vi "BioFeedback20(simple load data).vi"() -> ()   [LabVIEW 2016]
doc: "Use this template to build a producer/consumer design pattern. Use this template when you need to execute a process, such as data analysis, when a data source, such as a triggered acquisition, produces data at an uneven rate and you need to execute the process when the data becomes available."
uses:
  customSubVIs/8ChanWfmArray.ctl
  <vilib>/Utility/file.llb/Write Delimited Spreadsheet (string).vi
  <vilib>/Waveform/WDTFileIO.llb/Export Waveforms To Spreadsheet File (1D).vi
panel:
  in  "enableSave":bool caption="No Save      Save"
  in  "barOrGraph":bool=TRUE caption="Graph (under construction)       Bar"
  in  "Trial comment":string
  out "Collecting Data":bool
  in  "Display Min":dbl
  in  "Display Max":dbl=100.0
  in  "log filepath":path
  out "TrialStartTime":timestamp
  in  "Trial Duration (s)":dbl=3.0
  out "Trial Number":dbl
  in  "Session Name":string="Test"
  out "loopTime":dbl=30.0 caption="Upper Cut-Off"
  in  "trial display data":path
  out "Disp Data":cluster{"queue out":refnum<queue>, dbl, dbl}[](array[cluster])
  in  "Target Percentage":dbl=10.0
  out "DisplayActivation":dbl
  out "DisplayBarActivation":dbl(slide) caption="Percent Activation" max=1.0 scale=0.0..100.0
  in  "EMG Channel To Display":dbl=1.0
  out "MVC Data":cluster{"queue out":refnum<queue>, dbl, dbl}[](array[cluster])
  out "Trial Name":string="Test"
  in  "Data Directory":path=path "C:/Users/Tinggroup/Desktop/EMG Biofeedback System/LabviewFiles/Data"
  out "GetMaxStartTime":timestamp
  in  "MVC Number":dbl=1.0
  in  "SecondsToAcquireMax":dbl=3.0
  in  "Frames Per Second":dbl=30.0 caption="Upper Cut-Off"
  in  "EMG Input Device\nProduct Type":string="USB-6009"
  out "raw data":dynamicdata(graph)
  out "dispSize":dbl=20.0 caption="Lower Cut-Off"
  out "mvcSize":dbl=300.0 caption="Upper Cut-Off"
  in  "MVC Window Size (s)":dbl=0.5
  in  "Display Window Size (s)":dbl=0.5
  in  "MVC Raw Path":path
  in  "trial raw data":path
  in  "trial filtered data":path
  in  "MVC Filtered Path":path
  in  "Sample rate (Hz)":dbl=1000.0 caption="Upper Cut-Off"
  out "fps":dbl=20.0 caption="Lower Cut-Off"
  out "rate":dbl=300.0 caption="Upper Cut-Off"
  in  "Set Parameters":bool
  out "lower":dbl=20.0 caption="Lower Cut-Off"
  out "upper":dbl=300.0 caption="Upper Cut-Off"
  in  "Lower Cut-Off":dbl=20.0
  in  "Upper Cut-Off":dbl=500.0
  in  "Mark":bool
  in  "End Trial":bool
  in  "Reset MVC":bool
  in  "Get MVC":bool
  in  "StartTrial":bool
  out "State":T1(ring)
  out "FilteredAndRectified":waveform(dbl)[](graph) caption="Filtered and Rectified"
  in  "stop":bool
  # "Filtering"
  # "Add trial name\nBEFORE beginning trial"
  # "Display Settings"
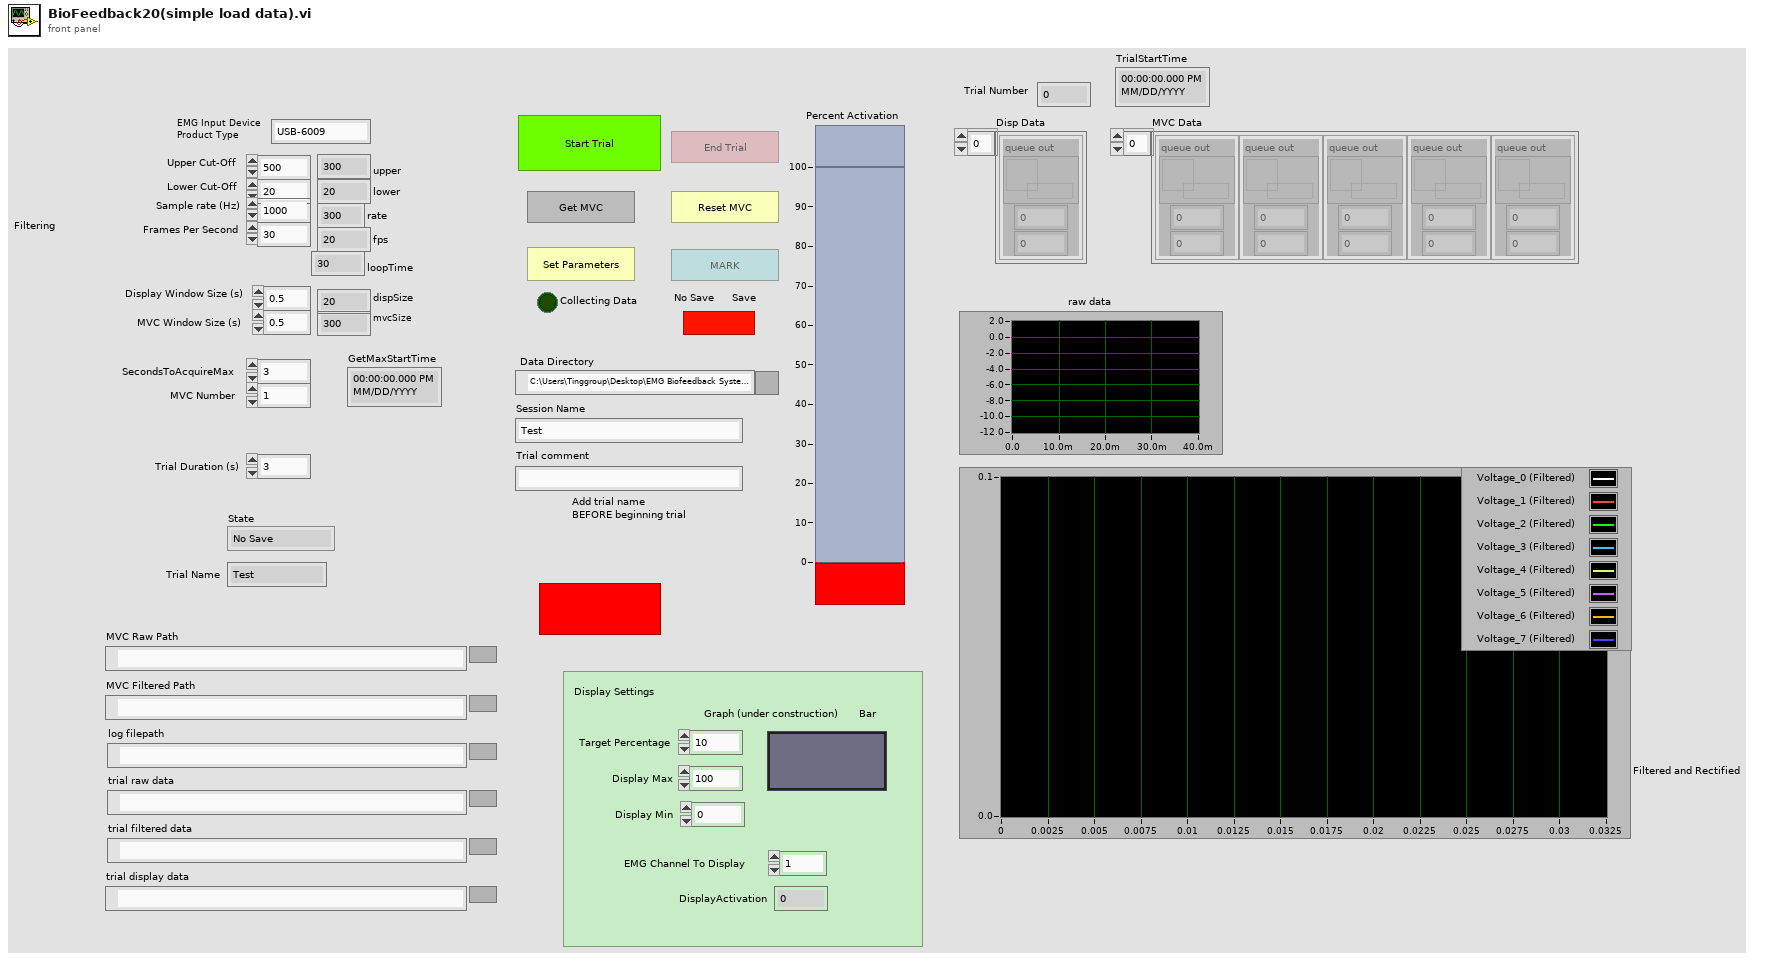
[diagram p1: front panel]
types:
  T1 = enum16{"No Save", "Acquiring Max", "Trial In Progress"}
  T2 = typedef "8ChanWfmArray.ctl" = waveform(dbl)[]
  T3 = enum8{"Enabled", "Disabled", "Disabled and Grayed Out"}
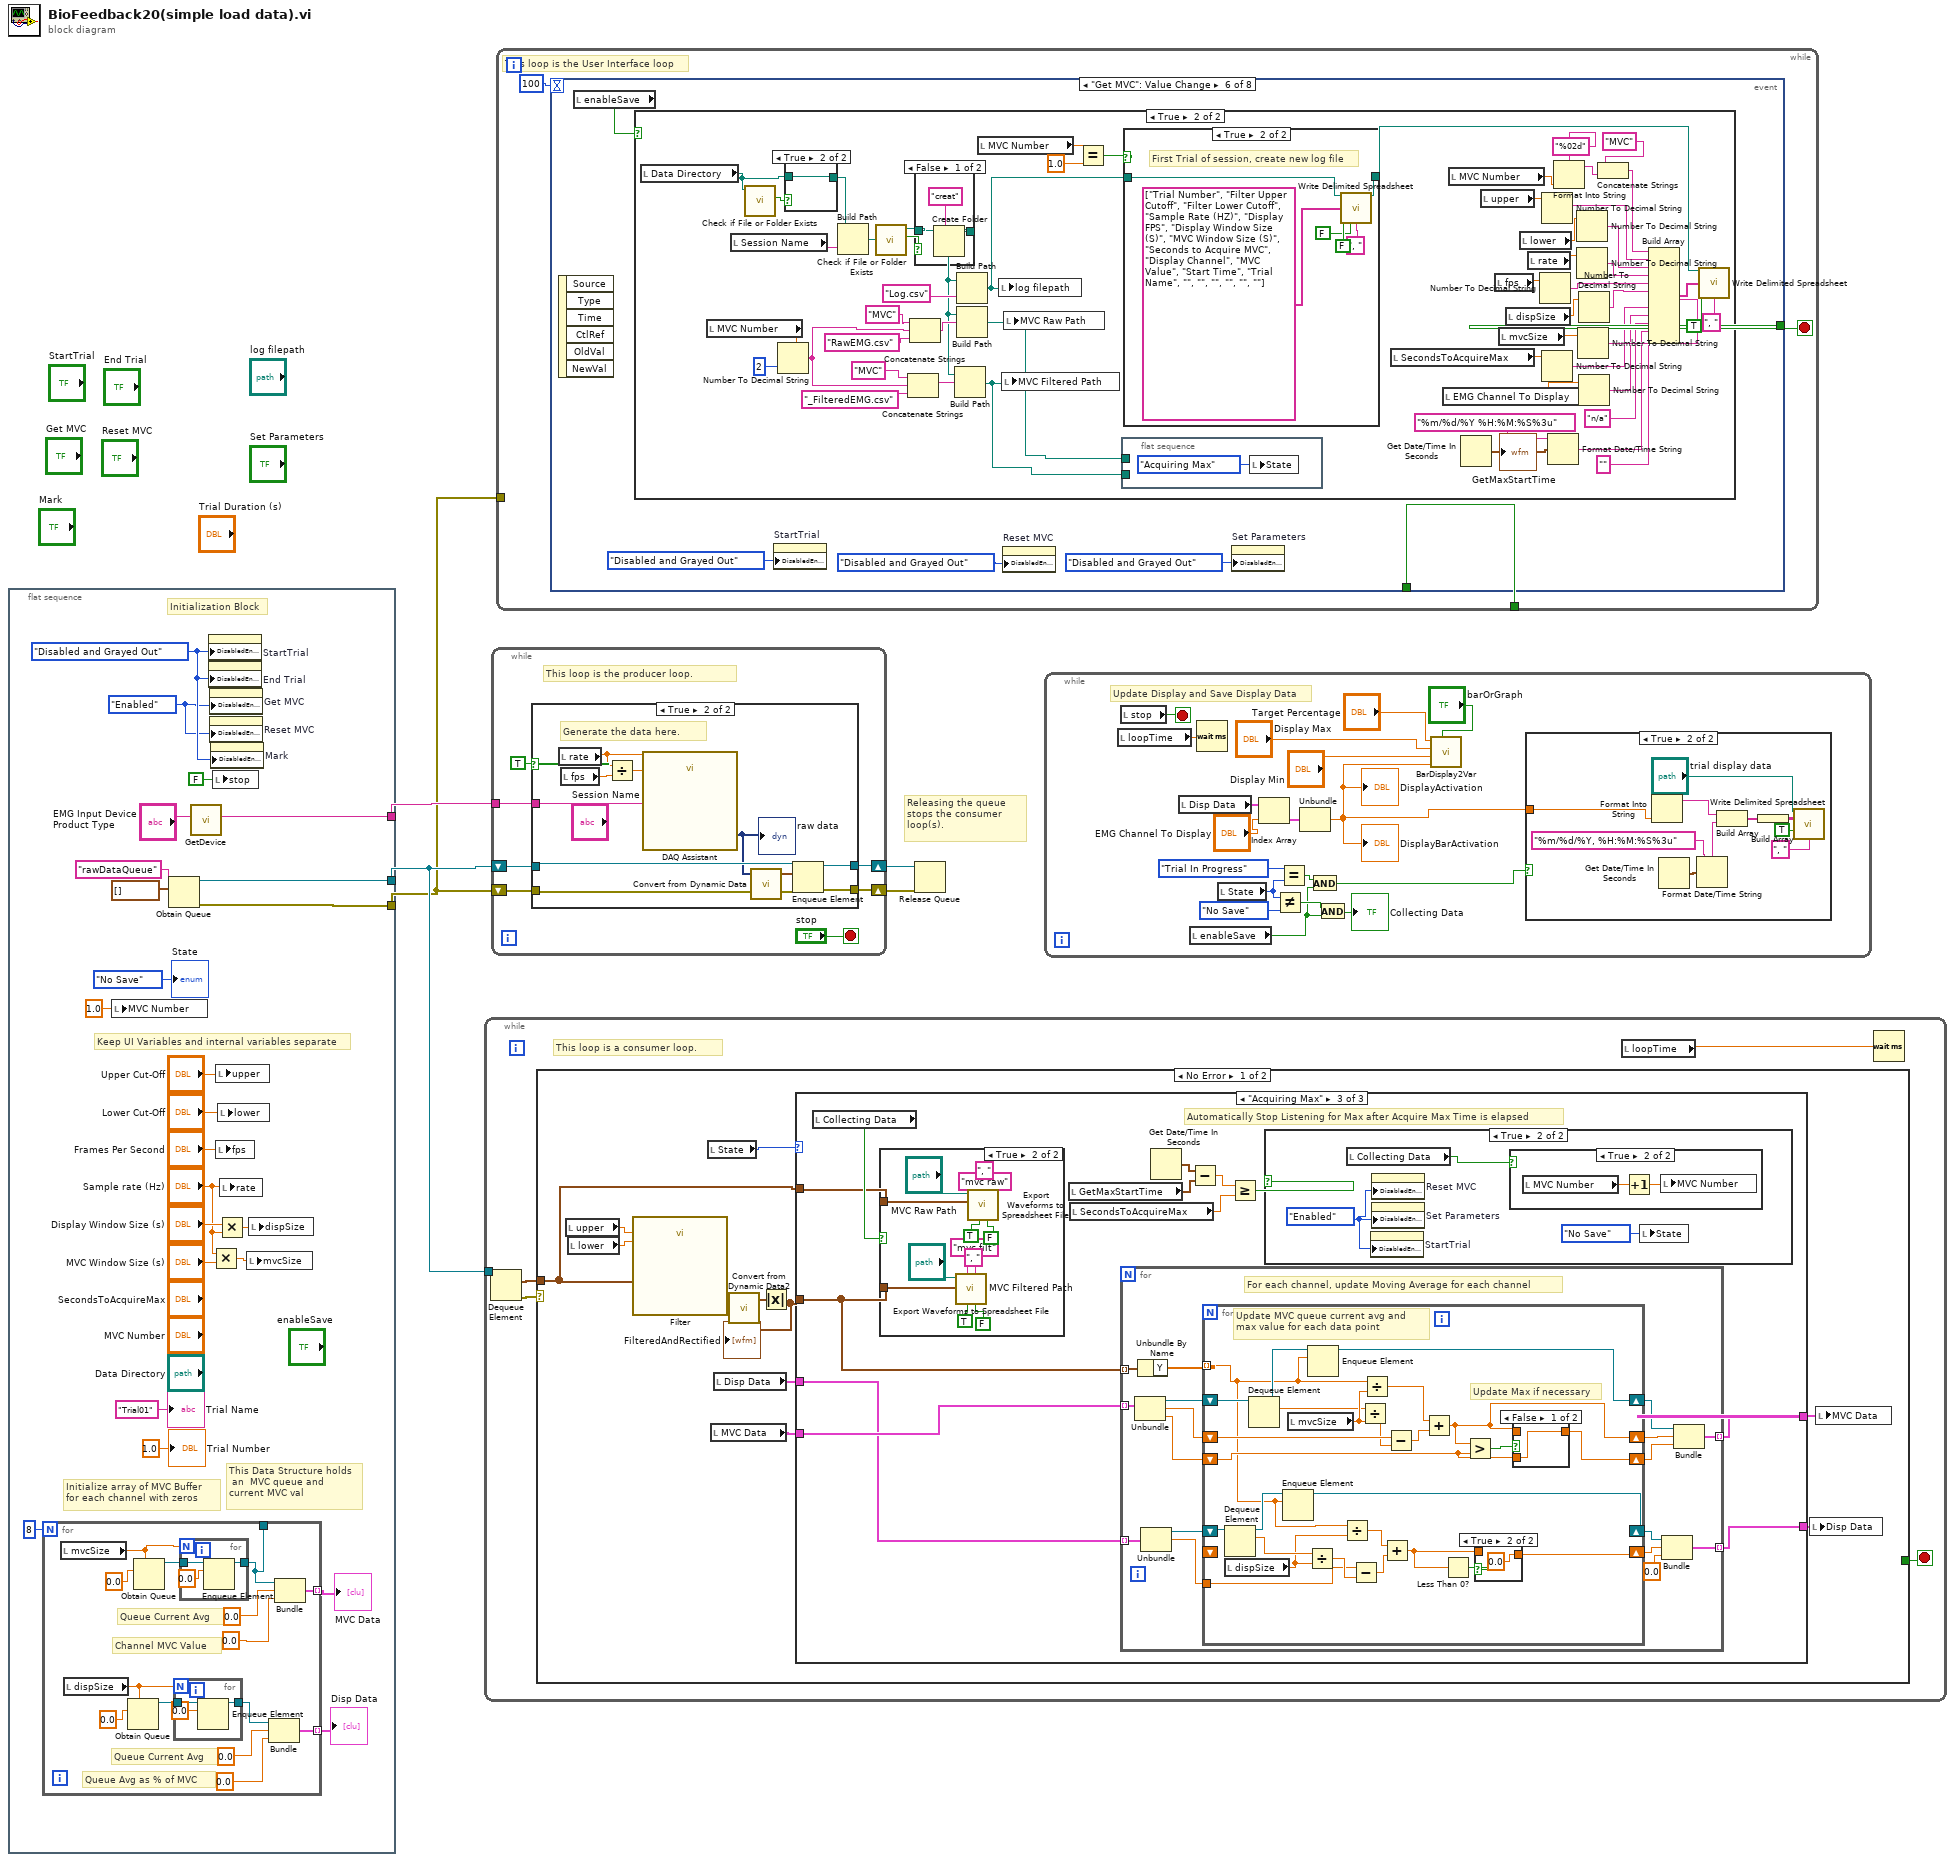
[diagram p0: block diagram]
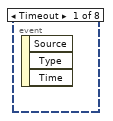
[diagram p3: hidden frame]
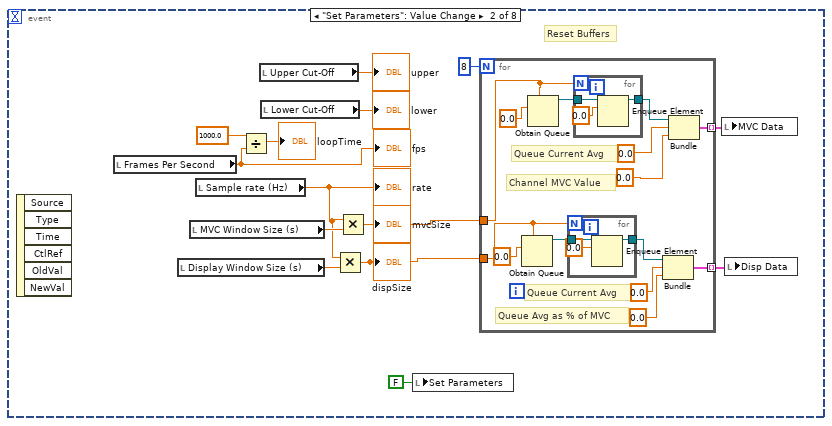
[diagram p4: hidden frame]
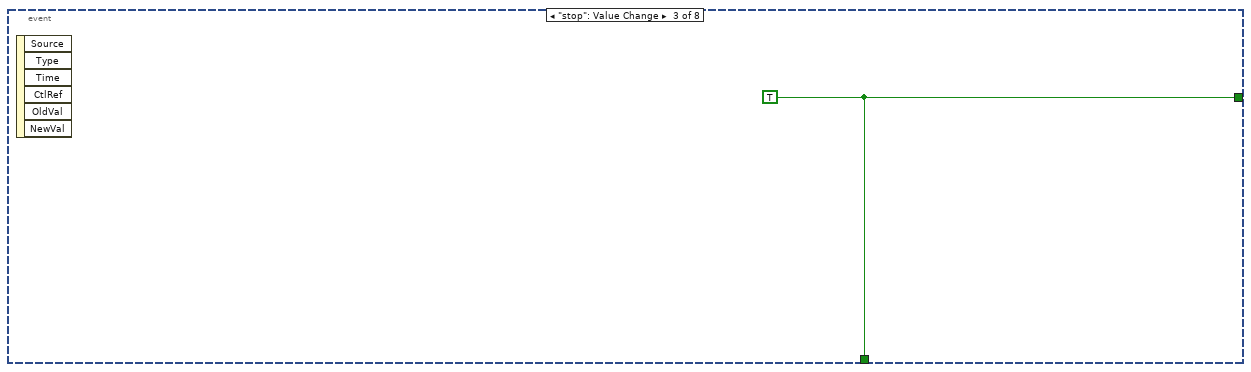
[diagram p5: hidden frame]
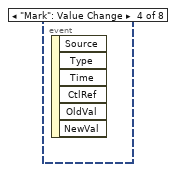
[diagram p6: hidden frame]
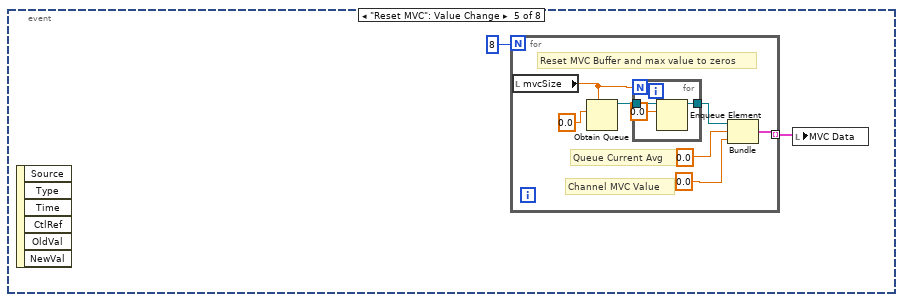
[diagram p7: hidden frame]
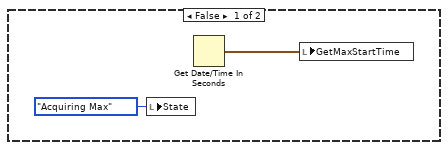
[diagram p8: hidden frame]
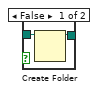
[diagram p11: hidden frame]
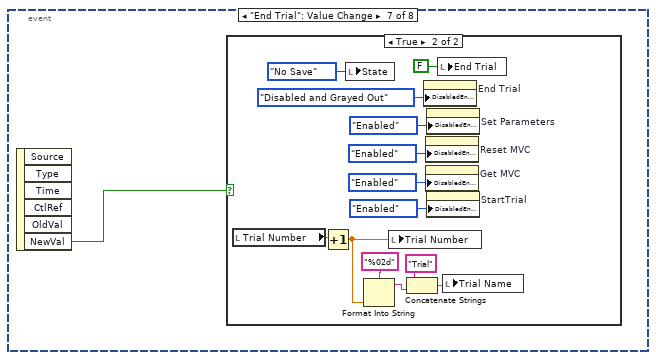
[diagram p12: hidden frame]
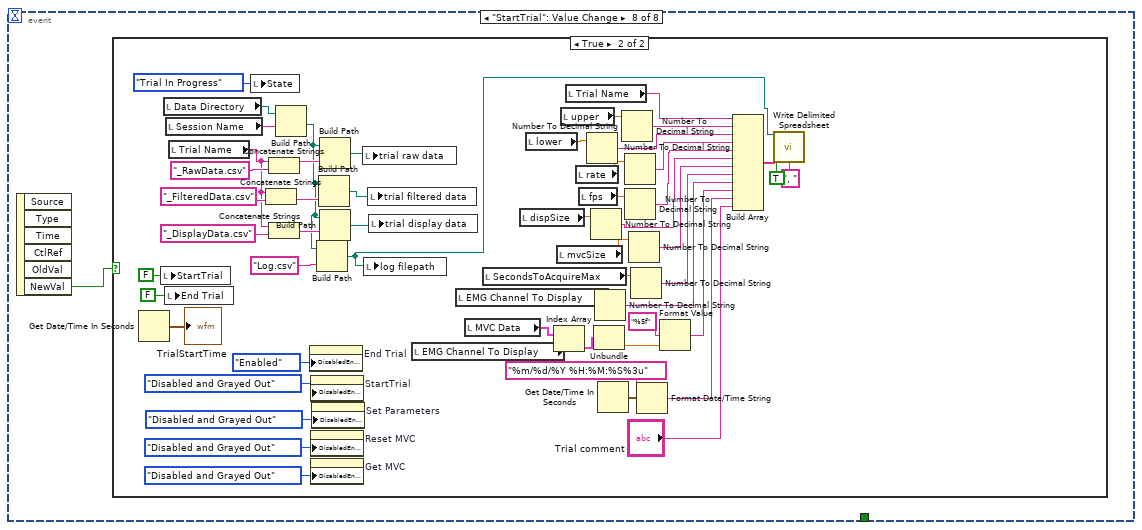
[diagram p14: hidden frame]
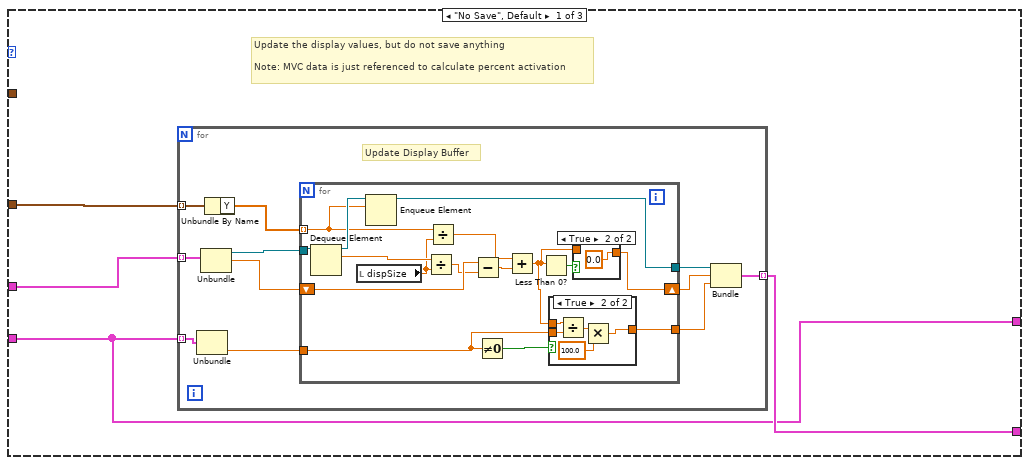
[diagram p16: hidden frame]
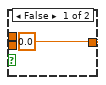
[diagram p18: hidden frame]
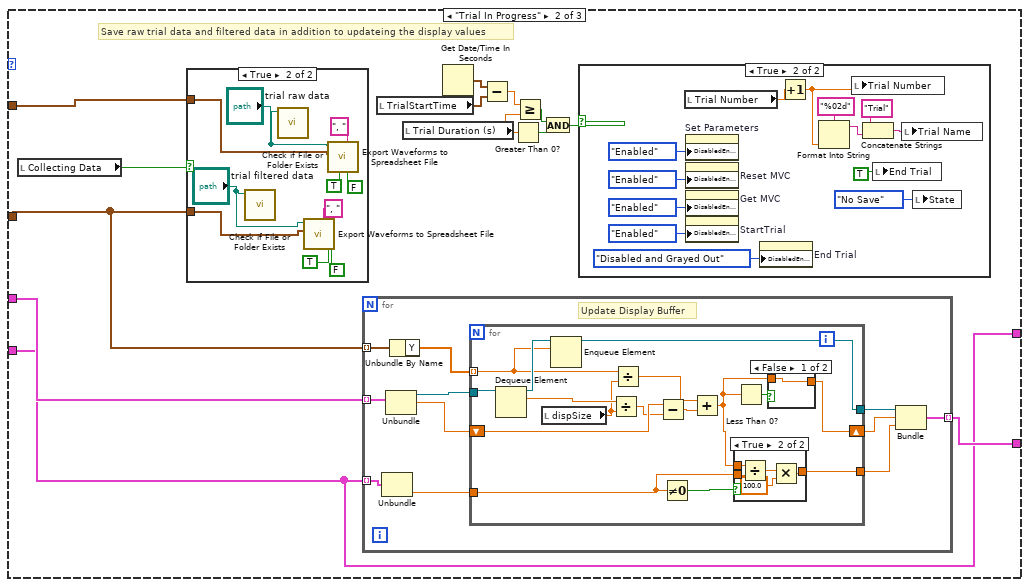
[diagram p19: hidden frame]
diagram:
  # "Releasing the queue stops the consumer loop(s)."
  n1 = flat-sequence {
    tunnel: [w20] -> w3
    tunnel: [w19] -> w2
    tunnel: [w22] -> w4
    frame #0 {
      w26 = T3."Enabled" ("Disabled")
      w27 = T3."Disabled and Grayed Out" ("Disabled")
      # "Keep UI Variables and internal variables separate"
      # "This Data Structure holds\n an  MVC queue and \ncurrent MVC val"
      # "Initialize array of MVC Buffer \nfor each channel with zeros"
      # "Initialization Block"
      n2 = for {
        N: 8 -> [_]
        tunnel: [w40] -> w12 mode=indexing
        tunnel: [w37] -> _
        tunnel: [w30] -> w11 mode=indexing
        # "Queue Avg as % of MVC"
        # "Queue Current Avg"
        # "Channel MVC Value"
        # "Queue Current Avg"
        n3 = local read "mvcSize"() -> (w41:dbl)
        n4 = local read "dispSize"() -> (w34:dbl)
        n5 = Obtain Queue(max queue size (-1, unlimited)=w34, element data type=0.0) -> (queue out=w31:refnum<queue>)  [unwired: 3 in, 2 out]
        n6 = Obtain Queue(max queue size (-1, unlimited)=w41, element data type=0.0) -> (queue out=w42:refnum<queue>)  [unwired: 3 in, 2 out]
        n7 = for {
          N: w34 -> [_]
          tunnel: w31 -> [w46]
          tunnel: [w44] -> w32
          n8 = Enqueue Element(queue=w46, element=0.0) -> (queue out=w44:refnum<queue>)  [unwired: 2 in, 2 out]
        }
        n9 = for {
          N: w41 -> [_]
          tunnel: w42 -> [w49]
          tunnel: [w47] -> w37
          n10 = Enqueue Element(queue=w49, element=0.0) -> (queue out=w47:refnum<queue>)  [unwired: 2 in, 2 out]
        }
        n11 = Bundle("queue out"=w32, 0.0, 0.0) -> (w30:cluster{"queue out":refnum<queue>, dbl, dbl})  [unwired: 1 in]
        n12 = Bundle("queue out"=w37, 0.0, 0.0) -> (w40:cluster{"queue out":refnum<queue>, dbl, dbl})  [unwired: 1 in]
      }
      "MVC Data" <- w12
      "Disp Data" <- w11
      n13 = local write "MVC Number"(1.0 ("MVC Number")) -> ()
      n14 = Obtain Queue(name (unnamed)="rawDataQueue", element data type=T2 [] ("initialized array")) -> (queue out=w20:refnum<queue>, error out=w19:errorcluster)  [unwired: 3 in, 1 out]
      n15 = call "GetDevice.vi"("EMG Input Device\nProduct Type"="EMG Input Device\nProduct Type") -> ("DAQmx Device Name"=w22:tag)  [unwired: 10 in]
      n16 = property on="StartTrial" class="Bool (strict)"("DisabledEnum"=w27) -> ()  [unwired: 2 in, 2 out]
      n17 = property on="End Trial" class="Bool (strict)"("DisabledEnum"=w27) -> ()  [unwired: 2 in, 2 out]
      n18 = property on="Get MVC" class="Bool"("DisabledEnum"=w26) -> ()  [unwired: 2 in, 2 out]
      n19 = property on="Reset MVC" class="Bool"("DisabledEnum"=w26) -> ()  [unwired: 2 in, 2 out]
      n20 = property on="Mark" class="Bool"("DisabledEnum"=w27) -> ()  [unwired: 2 in, 2 out]
      n21 = Multiply(x="Sample rate (Hz)", y="MVC Window Size (s)") -> (x*y=w14:dbl)
      n22 = local write "stop"(FALSE ("stop")) -> ()
      n23 = local write "upper"("Upper Cut-Off") -> ()
      n24 = local write "fps"("Frames Per Second") -> ()
      n25 = Multiply(x="Display Window Size (s)", y="Sample rate (Hz)") -> (x*y=w17:dbl)
      n26 = local write "lower"("Lower Cut-Off") -> ()
      n27 = local write "rate"("Sample rate (Hz)") -> ()
      n28 = local write "mvcSize"(w14) -> ()
      n29 = local write "dispSize"(w17) -> ()
      "Trial Name" <- "Trial01" ("Trial Name")
      "State" <- T1."No Save" ("State")
      "Trial Number" <- 1.0 ("Trial Number")
    }
  }
  n30 = while {
    tunnel: w3 -> [w51]
    stop <- w52 stop-if-true
    # "This loop is a consumer loop."
    n31 = Dequeue Element(queue=w51) -> (element=w53:T2, error out=w54:errorcluster)  [unwired: 2 in, 2 out]
    n32 = case shown="No Error" w54 {
      tunnel: w53 -> [w61 _]
      tunnel: [_ TRUE] -> w52
      frame No Error {
        n33 = local read "upper"() -> (w63:dbl)
        n34 = local read "lower"() -> (w62:dbl)
        n35 = call "Filter"("Lower Cut-Off"=w62, "Upper Cut-Off"=w63, "Signal"=w61) -> ("Filtered Signal"=w64:dynamicdata)  [unwired: 7 in, 1 out]
        n36 = local read "State"() -> (w55:T1)
        n37 = local read "MVC Data"() -> (w59:cluster{"queue out":refnum<queue>, dbl, dbl}[])
        n38 = local read "Disp Data"() -> (w58:cluster{"queue out":refnum<queue>, dbl, dbl}[])
        n39 = call "Convert from Dynamic Data2"("Dynamic Data Type"=w64) -> ("Array of Waveform"=w65:waveform(dbl)[])  [unwired: 3 in]
        n40 = Absolute Value(x=w65) -> (abs(x)=w60:waveform(dbl)[])
        "FilteredAndRectified" <- w60
        n41 = case shown="\"Acquiring Max\"" w55 {
          tunnel: w60 -> [w69 w107 w178]
          tunnel: w61 -> [_ w106 w179]
          tunnel: w59 -> [w66 w115 w182]
          tunnel: w58 -> [w68 w117 w181]
          tunnel: [w67 w116 w176] -> w56
          tunnel: [w66 w115 w177] -> w57
          frame "No Save", Default {
            # "Update the display values, but do not save anything\n\nNote: MVC data is just referenced to calculate percent activation"
            n42 = for {
              tunnel: w68 -> [w74] mode=indexing
              tunnel: w69 -> [w79] mode=indexing
              tunnel: [w75] -> w67 mode=indexing
              tunnel: w66 -> [w72] mode=indexing
              # "Update Display Buffer"
              n43 = Unbundle(w72) -> (w71:dbl)  [unwired: 2 out]
              n44 = Unbundle(w74) -> ("queue out"=w80:refnum<queue>, w73:dbl)  [unwired: 1 out]
              n45 = Unbundle By Name(w79) -> ("Y"=w78:dbl[])
              n46 = for {
                tunnel: w80 -> [w90]
                tunnel: w78 -> [w86] mode=indexing
                shift-right: [w83] -> w77
                shift-left: w73 -> [w95]
                tunnel: [w85] -> w76
                tunnel: w71 -> [w88]
                tunnel: [w84] -> w70
                n47 = Dequeue Element(queue=w90) -> (queue out=w87:refnum<queue>, element=w96:dbl)  [unwired: 2 in, 2 out]
                n48 = local read "dispSize"() -> (w93:dbl)
                n49 = Enqueue Element(queue=w87, element=w86) -> (queue out=w85:refnum<queue>)  [unwired: 2 in, 2 out]
                n50 = Divide(x=w96, y=w93) -> (x/y=w94:dbl)
                n51 = Divide(x=w86, y=w93) -> (x/y=w91:dbl)
                n52 = Subtract(x=w95, y=w94) -> (x-y=w92:dbl)
                n53 = Not Equal To 0?(x=w88) -> (x != 0?=w89:bool)
                n54 = Add(x=w91, y=w92) -> (x+y=w81:dbl)
                n55 = Less Than 0?(x=w81) -> (x < 0?=w82:bool)
                n56 = case shown="True" w89 {
                  tunnel: w88 -> [_ w104]
                  tunnel: [0.0 w100] -> w84
                  tunnel: w81 -> [_ w103]
                  frame False {
                  }
                  frame True {
                    n57 = Divide(x=w103, y=w104) -> (x/y=w101:dbl)
                    n58 = Multiply(x=w101, y=100.0) -> (x*y=w100:dbl)
                  }
                }
                n59 = case shown="True" w82 {
                  tunnel: [w97 0.0] -> w83
                  tunnel: w81 -> [w97 _]
                  frame False {
                  }
                  frame True {
                  }
                }
              }
              n60 = Bundle("queue out"=w76, w77, w70) -> (w75:cluster{"queue out":refnum<queue>, dbl, dbl})  [unwired: 1 in]
            }
          }
          frame "Trial In Progress" {
            # "Save raw trial data and filtered data in addition to updateing the display values"
            n61 = local read "Collecting Data"() -> (w105:bool)
            n62 = case shown="True" w105 {
              tunnel: w107 -> [_ w122]
              tunnel: w106 -> [_ w120]
              frame False {
              }
              frame True {
                n63 = call <vilib>:"Check if File or Folder Exists.vi"("path"="trial filtered data") -> ()  [unwired: 8 in, 3 out]
                n64 = call <vilib>:"Check if File or Folder Exists.vi"("path"="trial raw data") -> ()  [unwired: 8 in, 3 out]
                n65 = call-poly <vilib>:"Export Waveforms to Spreadsheet File.vi"("header? (write header:T)"=FALSE, "delimiter (Tab)"=", ", "append to file? (new file:F)"=TRUE, "waveforms"=w122, "file path (dialog if empty)"="trial filtered data") -> ()  [unwired: 5 in, 2 out]
                n66 = call-poly <vilib>:"Export Waveforms to Spreadsheet File.vi"("header? (write header:T)"=FALSE, "delimiter (Tab)"=", ", "append to file? (new file:F)"=TRUE, "waveforms"=w120, "file path (dialog if empty)"="trial raw data") -> ()  [unwired: 5 in, 2 out]
              }
            }
            n67 = for {
              tunnel: w117 -> [w145] mode=indexing
              tunnel: w107 -> [w150] mode=indexing
              tunnel: [w146] -> w116 mode=indexing
              tunnel: w115 -> [w143] mode=indexing
              # "Update Display Buffer"
              n68 = Unbundle(w143) -> (w142:dbl)  [unwired: 2 out]
              n69 = Unbundle(w145) -> ("queue out"=w151:refnum<queue>, w144:dbl)  [unwired: 1 out]
              n70 = Unbundle By Name(w150) -> ("Y"=w149:dbl[])
              n71 = for {
                tunnel: w151 -> [w161]
                tunnel: w149 -> [w157] mode=indexing
                shift-right: [w152] -> w148
                shift-left: w144 -> [w166]
                tunnel: [w156] -> w147
                tunnel: w142 -> [w159]
                tunnel: [w155] -> w141
                n72 = Dequeue Element(queue=w161) -> (queue out=w158:refnum<queue>, element=w167:dbl)  [unwired: 2 in, 2 out]
                n73 = local read "dispSize"() -> (w164:dbl)
                n74 = Enqueue Element(queue=w158, element=w157) -> (queue out=w156:refnum<queue>)  [unwired: 2 in, 2 out]
                n75 = Divide(x=w167, y=w164) -> (x/y=w165:dbl)
                n76 = Divide(x=w157, y=w164) -> (x/y=w162:dbl)
                n77 = Subtract(x=w166, y=w165) -> (x-y=w163:dbl)
                n78 = Not Equal To 0?(x=w159) -> (x != 0?=w160:bool)
                n79 = Add(x=w162, y=w163) -> (x+y=w153:dbl)
                n80 = case shown="True" w160 {
                  tunnel: w159 -> [_ w175]
                  tunnel: [0.0 w173] -> w155
                  tunnel: w153 -> [_ w174]
                  frame False {
                  }
                  frame True {
                    n81 = Divide(x=w174, y=w175) -> (x/y=w172:dbl)
                    n82 = Multiply(x=w172, y=100.0) -> (x*y=w173:dbl)
                  }
                }
                n83 = Less Than 0?(x=w153) -> (x < 0?=w154:bool)
                n84 = case shown="False" w154 {
                  tunnel: [w168 0.0] -> w152
                  tunnel: w153 -> [w168 _]
                  frame False {
                  }
                  frame True {
                  }
                }
              }
              n85 = Bundle("queue out"=w147, w148, w141) -> (w146:cluster{"queue out":refnum<queue>, dbl, dbl})  [unwired: 1 in]
            }
            n86 = local read "TrialStartTime"() -> (w113:timestamp)
            n87 = local read "Trial Duration (s)"() -> (w109:dbl)
            n88 = Get Date/Time In Seconds() -> (seconds since 1Jan1904=w112:timestamp)
            n89 = Subtract(x=w112, y=w113) -> (x-y=w114:dbl)
            n90 = Greater Than 0?(x=w109) -> (x > 0?=w110:bool)
            n91 = Greater Or Equal?(x=w114, y=w109) -> (x >= y?=w108:bool)
            n92 = And(x=w108, y=w110) -> (x .and. y?=w111:bool)
            n93 = case shown="True" w111 {
              frame False {
              }
              frame True {
                n94 = local read "Trial Number"() -> (w129:dbl)
                n95 = property on="Set Parameters" class="Bool (strict)"("DisabledEnum"=T3."Enabled" ("Disabled")) -> ()  [unwired: 2 in, 2 out]
                n96 = property on="Reset MVC" class="Bool"("DisabledEnum"=T3."Enabled" ("Disabled")) -> ()  [unwired: 2 in, 2 out]
                n97 = property on="Get MVC" class="Bool"("DisabledEnum"=T3."Enabled" ("Disabled")) -> ()  [unwired: 2 in, 2 out]
                n98 = property on="StartTrial" class="Bool (strict)"("DisabledEnum"=T3."Enabled" ("Disabled")) -> ()  [unwired: 2 in, 2 out]
                n99 = property on="End Trial" class="Bool (strict)"("DisabledEnum"=T3."Disabled and Grayed Out" ("Disabled")) -> ()  [unwired: 2 in, 2 out]
                n100 = Increment(x=w129) -> (x+1=w128:dbl)
                n101 = Format Into String(format string="%02d", w128) -> (resulting string=w135:string)  [unwired: 2 in, 1 out]
                n102 = local write "Trial Number"(w128) -> ()
                n103 = Concatenate Strings("Trial" ("string"), w135) -> (w139:string)
                n104 = local write "End Trial"(TRUE ("End Trial")) -> ()
                n105 = local write "Trial Name"(w139) -> ()
                n106 = local write "State"(T1."No Save" ("State")) -> ()
              }
            }
          }
          frame "Acquiring Max" {
            # "Automatically Stop Listening for Max after Acquire Max Time is elapsed"
            n107 = local read "Collecting Data"() -> (w180:bool)
            n108 = case shown="True" w180 {
              tunnel: w179 -> [_ w194]
              tunnel: w178 -> [_ w193]
              frame False {
              }
              frame True {
                n109 = call-poly <vilib>:"Export Waveforms to Spreadsheet File.vi"("header? (write header:T)"=FALSE, "delimiter (Tab)"=", ", "append to file? (new file:F)"=TRUE, "prompt"="mvc filt", "waveforms"=w193, "file path (dialog if empty)"="MVC Filtered Path") -> ()  [unwired: 4 in, 2 out]
                n110 = call-poly <vilib>:"Export Waveforms to Spreadsheet File.vi"("header? (write header:T)"=FALSE, "delimiter (Tab)"=", ", "append to file? (new file:F)"=TRUE, "prompt"="mvc raw", "waveforms"=w194, "file path (dialog if empty)"="MVC Raw Path") -> ()  [unwired: 4 in, 2 out]
              }
            }
            n111 = local read "GetMaxStartTime"() -> (w186:timestamp)
            n112 = local read "SecondsToAcquireMax"() -> (w184:dbl)
            n113 = for {
              tunnel: w178 -> [w221] mode=indexing
              tunnel: w182 -> [w219] mode=indexing
              tunnel: [w213] -> w177 mode=indexing
              tunnel: w181 -> [w211] mode=indexing
              tunnel: [w205] -> w176 mode=indexing
              # "For each channel, update Moving Average for each channel"
              n114 = Unbundle(w219) -> ("queue out"=w212:refnum<queue>, w218:dbl, w217:dbl)
              n115 = Unbundle By Name(w221) -> ("Y"=w220:dbl[])
              n116 = Unbundle(w211) -> ("queue out"=w207:refnum<queue>, w210:dbl)  [unwired: 1 out]
              n117 = for {
                tunnel: w220 -> [w230] mode=indexing
                shift-right: [w235] -> w215
                shift-left: w218 -> [w247]
                shift-right: [w239] -> w216
                shift-left: w212 -> [w238]
                shift-right: [w241] -> w214
                shift-left: w217 -> [w240]
                tunnel: w210 -> [w228]
                shift-right: [w223] -> w208
                shift-left: _ -> [_]
                shift-right: [w232] -> w209
                shift-left: w207 -> [w225]
                # "Update Max if necessary"
                # "Update MVC queue current avg and \nmax value for each data point"
                n118 = Dequeue Element(queue=w225) -> (queue out=w234:refnum<queue>, element=w233:dbl)  [unwired: 2 in, 2 out]
                n119 = local read "dispSize"() -> (w231:dbl)
                n120 = Dequeue Element(queue=w238) -> (queue out=w237:refnum<queue>, element=w236:dbl)  [unwired: 2 in, 2 out]
                n121 = Enqueue Element(queue=w234, element=w230) -> (queue out=w232:refnum<queue>)  [unwired: 2 in, 2 out]
                n122 = local read "mvcSize"() -> (w245:dbl)
                n123 = Divide(x=w233, y=w231) -> (x/y=w229:dbl)
                n124 = Enqueue Element(queue=w237, element=w230) -> (queue out=w239:refnum<queue>)  [unwired: 2 in, 2 out]
                n125 = Divide(x=w230, y=w231) -> (x/y=w227:dbl)
                n126 = Subtract(x=w228, y=w229) -> (x-y=w226:dbl)
                n127 = Divide(x=w236, y=w245) -> (x/y=w246:dbl)
                n128 = Divide(x=w230, y=w245) -> (x/y=w243:dbl)
                n129 = Add(x=w227, y=w226) -> (x+y=w222:dbl)
                n130 = Subtract(x=w247, y=w246) -> (x-y=w244:dbl)
                n131 = Add(x=w243, y=w244) -> (x+y=w235:dbl)
                n132 = Less Than 0?(x=w222) -> (x < 0?=w224:bool)
                n133 = Greater?(x=w235, y=w240) -> (0:w242:bool)
                n134 = case shown="True" w224 {
                  tunnel: [w248 0.0] -> w223
                  tunnel: w222 -> [w248 _]
                  frame False {
                  }
                  frame True {
                  }
                }
                n135 = case shown="False" w242 {
                  tunnel: w235 -> [_ w251]
                  tunnel: [w250 w251] -> w241
                  tunnel: w240 -> [w250 _]
                  frame False {
                  }
                  frame True {
                  }
                }
              }
              n136 = Bundle("queue out"=w209, w208, 0.0) -> (w205:cluster{"queue out":refnum<queue>, dbl, dbl})  [unwired: 1 in]
              n137 = Bundle("queue out"=w216, w215, w214) -> (w213:cluster{"queue out":refnum<queue>, dbl, dbl})  [unwired: 1 in]
            }
            n138 = Get Date/Time In Seconds() -> (seconds since 1Jan1904=w187:timestamp)
            n139 = Subtract(x=w187, y=w186) -> (x-y=w185:dbl)
            n140 = Greater Or Equal?(x=w185, y=w184) -> (x >= y?=w183:bool)
            n141 = case shown="True" w183 {
              frame False {
              }
              frame True {
                w201 = T3."Enabled" ("Disabled")
                n142 = local read "Collecting Data"() -> (w200:bool)
                n143 = property on="StartTrial" class="Bool (strict)"("DisabledEnum"=w201) -> ()  [unwired: 2 in, 2 out]
                n144 = property on="Reset MVC" class="Bool"("DisabledEnum"=w201) -> ()  [unwired: 2 in, 2 out]
                n145 = property on="Set Parameters" class="Bool (strict)"("DisabledEnum"=w201) -> ()  [unwired: 2 in, 2 out]
                n146 = case shown="True" w200 {
                  frame False {
                  }
                  frame True {
                    n147 = local read "MVC Number"() -> (w204:dbl)
                    n148 = Increment(x=w204) -> (x+1=w203:dbl)
                    n149 = local write "MVC Number"(w203) -> ()
                  }
                }
                n150 = local write "State"(T1."No Save" ("State")) -> ()
              }
            }
          }
        }
        n151 = local write "Disp Data"(w56) -> ()
        n152 = local write "MVC Data"(w57) -> ()
      }
      frame Error {
        # "Return true for any case which should stop the loop."
      }
    }
    n153 = local read "loopTime"() -> (w50:dbl)
    n154 = Wait (ms)(milliseconds to wait=w50) -> ()  [unwired: 1 out]
  }
  n155 = while {
    shift-right: [w255] -> w1
    shift-left: w2 -> [w256]
    shift-right: [w257] -> w5
    shift-left: w3 -> [w258]
    tunnel: w4 -> [w253]
    stop <- "stop" stop-if-true
    # "This loop is the producer loop."
    n156 = case shown="True" TRUE ("Case Constant\n(See Context Help)") {
      tunnel: w258 -> [w261 w271]
      tunnel: [w261 w270] -> w257
      tunnel: w256 -> [w260 w269]
      tunnel: [w260 w268] -> w255
      tunnel: w253 -> [_ w262]
      frame False {
      }
      frame True {
        # "Generate the data here."
        n157 = local read "rate"() -> (w265:dbl)
        n158 = local read "fps"() -> (w266:dbl)
        n159 = Divide(x=w265, y=w266) -> (x/y=w264:dbl)
        n160 = call "DAQ Assistant"("rate"=w265, "number of samples"=w264, "device name"=w262) -> ("data"=w263:dynamicdata)  [unwired: 13 in, 3 out]
        "raw data" <- w263
        n161 = call "Convert from Dynamic Data"("Dynamic Data Type"=w263) -> ("Array of Waveform"=w267:waveform(dbl)[])  [unwired: 3 in]
        n162 = Enqueue Element(queue=w271, element=w267, error in (no error)=w269) -> (queue out=w270:refnum<queue>, error out=w268:errorcluster)  [unwired: 1 in, 1 out]
      }
    }
  }
  n163 = while {
    tunnel: [w274] -> _
    tunnel: w2 -> [_]
    stop <- w272 stop-if-true
    # "This loop is the User Interface loop"
    n164 = event shown="[5] \"Get MVC\": Value Change" {
      selector: _ -> [_ _ _ _ _ _ _ _]
      dyn-events: _ -> [_ _ _ _ _ _ _ _]
      timeout: u32 100 ("milliseconds to wait") -> [_ _ _ _ _ _ _ _]
      tunnel: [_ _ w309 _ _ _ _ _] -> w272
      tunnel: [_ _ w309 _ _ _ _ _] -> w274
      event Timeout {
        n165 = event-data() -> ()  [unwired: 1 in, 3 out]
      }
      event "Set Parameters": Value Change {
        # "Reset Buffers"
        n166 = event-data() -> ()  [unwired: 1 in, 6 out]
        n167 = local read "Frames Per Second"() -> (w276:dbl)
        "fps" <- w276
        n168 = local read "Display Window Size (s)"() -> (w286:dbl)
        n169 = local read "MVC Window Size (s)"() -> (w287:dbl)
        n170 = local read "Sample rate (Hz)"() -> (w284:dbl)
        "rate" <- w284
        n171 = Divide(x=1000.0, y=w276) -> (x/y=→"loopTime":dbl)
        n172 = local read "Upper Cut-Off"() -> (→"upper":dbl)
        n173 = local read "Lower Cut-Off"() -> (→"lower":dbl)
        n174 = Multiply(x=w284, y=w286) -> (x*y=w282:dbl)
        "dispSize" <- w282
        n175 = Multiply(x=w284, y=w287) -> (x*y=w283:dbl)
        "mvcSize" <- w283
        n176 = local write "Set Parameters"(FALSE ("Set Parameters")) -> ()
        n177 = for {
          N: 8 -> [_]
          tunnel: [w300] -> w280 mode=indexing
          tunnel: [w291] -> w281 mode=indexing
          tunnel: w283 -> [w290]
          tunnel: w282 -> [w289]
          # "Queue Avg as % of MVC"
          # "Queue Current Avg"
          # "Channel MVC Value"
          # "Queue Current Avg"
          n178 = Obtain Queue(max queue size (-1, unlimited)=w289, element data type=0.0) -> (queue out=w292:refnum<queue>)  [unwired: 3 in, 2 out]
          n179 = Obtain Queue(max queue size (-1, unlimited)=w290, element data type=0.0) -> (queue out=w301:refnum<queue>)  [unwired: 3 in, 2 out]
          n180 = for {
            N: w289 -> [_]
            tunnel: w292 -> [w305]
            tunnel: [w303] -> w293
            n181 = Enqueue Element(queue=w305, element=0.0) -> (queue out=w303:refnum<queue>)  [unwired: 2 in, 2 out]
          }
          n182 = for {
            N: w290 -> [_]
            tunnel: w301 -> [w308]
            tunnel: [w306] -> w297
            n183 = Enqueue Element(queue=w308, element=0.0) -> (queue out=w306:refnum<queue>)  [unwired: 2 in, 2 out]
          }
          n184 = Bundle("queue out"=w293, 0.0, 0.0) -> (w291:cluster{"queue out":refnum<queue>, dbl, dbl})  [unwired: 1 in]
          n185 = Bundle("queue out"=w297, 0.0, 0.0) -> (w300:cluster{"queue out":refnum<queue>, dbl, dbl})  [unwired: 1 in]
        }
        n186 = local write "MVC Data"(w280) -> ()
        n187 = local write "Disp Data"(w281) -> ()
      }
      event "stop": Value Change {
        w309 = TRUE
        n188 = event-data() -> ()  [unwired: 1 in, 6 out]
      }
      event "Mark": Value Change {
        n189 = event-data() -> ()  [unwired: 1 in, 6 out]
      }
      event "Reset MVC": Value Change {
        n190 = event-data() -> ()  [unwired: 1 in, 6 out]
        n191 = for {
          N: 8 -> [_]
          tunnel: [w312] -> w311 mode=indexing
          # "Channel MVC Value"
          # "Queue Current Avg"
          # "Reset MVC Buffer and max value to zeros"
          n192 = local read "mvcSize"() -> (w315:dbl)
          n193 = Obtain Queue(max queue size (-1, unlimited)=w315, element data type=0.0) -> (queue out=w314:refnum<queue>)  [unwired: 3 in, 2 out]
          n194 = for {
            N: w315 -> [_]
            tunnel: w314 -> [w321]
            tunnel: [w319] -> w316
            n195 = Enqueue Element(queue=w321, element=0.0) -> (queue out=w319:refnum<queue>)  [unwired: 2 in, 2 out]
          }
          n196 = Bundle("queue out"=w316, 0.0, 0.0) -> (w312:cluster{"queue out":refnum<queue>, dbl, dbl})  [unwired: 1 in]
        }
        n197 = local write "MVC Data"(w311) -> ()
      }
      event "Get MVC": Value Change {
        n198 = event-data() -> ()  [unwired: 1 in, 6 out]
        n199 = local read "enableSave"() -> (w322:bool)
        n200 = case shown="True" w322 {
          frame False {
            n201 = local write "State"(T1."Acquiring Max" ("State")) -> ()
            n202 = Get Date/Time In Seconds() -> (seconds since 1Jan1904=w326:timestamp)
            n203 = local write "GetMaxStartTime"(w326) -> ()
          }
          frame True {
            n204 = local read "Data Directory"() -> (w330:path)
            n205 = local read "MVC Number"() -> (w375:dbl)
            n206 = local read "Session Name"() -> (w374:string)
            n207 = call <vilib>:"Check if File or Folder Exists.vi"("path"=w330) -> ("file or folder exists?"=w331:bool)  [unwired: 8 in, 2 out]
            n208 = Number To Decimal String(number=w375, width (-)=i16 2) -> (decimal integer string=w356:string)
            n209 = case shown="True" w331 {
              tunnel: [w395 w396] -> w370
              tunnel: w330 -> [w394 w396]
              frame False {
                n210 = Create Folder(path (use dialog)=w394) -> (created path=w395:path)  [unwired: 2 in, 2 out]
              }
              frame True {
              }
            }
            n211 = Build Path(base path=w370, name or relative path=w374) -> (appended path=w373:path)
            n212 = call <vilib>:"Check if File or Folder Exists.vi"("path"=w373) -> ("file or folder exists?"=w372:bool, "dup path"=w371:path)  [unwired: 8 in, 1 out]
            n213 = Concatenate Strings("MVC" ("string"), w356, "_FilteredEMG.csv" ("string")) -> (w380:string)
            n214 = Concatenate Strings("MVC" ("string"), w356, "RawEMG.csv" ("string")) -> (w379:string)
            n215 = case shown="False" w372 {
              tunnel: w371 -> [w392 w393]
              tunnel: [w391 w393] -> w367
              frame False {
                n216 = Create Folder(prompt (Create Folder)="creat", path (use dialog)=w392) -> (created path=w391:path)  [unwired: 1 in, 2 out]
              }
              frame True {
              }
            }
            n217 = Build Path(base path=w367, name or relative path=w380) -> (appended path=w328:path)
            n218 = Build Path(base path=w367, name or relative path="Log.csv" ("string")) -> (appended path=w344:path)
            n219 = Build Path(base path=w367, name or relative path=w379) -> (appended path=w329:path)
            n220 = local read "MVC Number"() -> (w347:dbl)
            n221 = local write "log filepath"(w344) -> ()
            n222 = local write "MVC Filtered Path"(w328) -> ()
            n223 = local write "MVC Raw Path"(w329) -> ()
            n224 = Equal?(x=w347, y=1.0) -> (x = y?=w337:bool)
            n225 = flat-sequence {
              tunnel: w329 -> [_]
              tunnel: w328 -> [_]
              frame #0 {
                n226 = local write "State"(T1."Acquiring Max" ("State")) -> ()
              }
            }
            n227 = case shown="True" w337 {
              tunnel: [w383 w387] -> w345
              tunnel: w344 -> [w383 w384]
              frame False {
                # "Do not create a new log file, use existing \nlog file"
              }
              frame True {
                # "First Trial of session, create new log file"
                n228 = call-poly <vilib>:"Write Delimited Spreadsheet.vi"("file path (dialog if empty)"=w384, "1D data"=string[] ["Trial Number", "Filter Upper Cutoff", "Filter Lower Cutoff", "Sample Rate (HZ)", "Display FPS", "Display Window Size (S)", "MVC Window Size (S)", "Seconds to Acquire MVC", "Display Channel", "MVC Value", "Start Time", "Trial Name", "", "", "", "", "", ""], "append to file? (new file:F)"=FALSE, "transpose? (no:F)"=FALSE, "delimiter (\\t)"=", " ("delimiter (\\t)")) -> ("new file path (Not A Path if cancelled)"=w387:path)  [unwired: 9 in, 1 out]
              }
            }
            n229 = local read "SecondsToAcquireMax"() -> (w361:dbl)
            n230 = local read "EMG Channel To Display"() -> (w360:dbl)
            n231 = local read "MVC Number"() -> (w340:dbl)
            n232 = Get Date/Time In Seconds() -> (seconds since 1Jan1904=w335:timestamp)
            "GetMaxStartTime" <- w335
            n233 = local read "upper"() -> (w366:dbl)
            n234 = local read "fps"() -> (w363:dbl)
            n235 = local read "mvcSize"() -> (w362:dbl)
            n236 = local read "dispSize"() -> (w357:dbl)
            n237 = local read "lower"() -> (w365:dbl)
            n238 = local read "rate"() -> (w364:dbl)
            n239 = Number To Decimal String(number=w363) -> (decimal integer string=w353:string)  [unwired: 1 in]
            n240 = Number To Decimal String(number=w366) -> (decimal integer string=w338:string)  [unwired: 1 in]
            n241 = Number To Decimal String(number=w361) -> (decimal integer string=w350:string)  [unwired: 1 in]
            n242 = Format Date/Time String(time format string (%c)="%m/%d/%Y %H:%M:%S%3u", seconds (now)=w335) -> (date/time string=w333:string)  [unwired: 1 in]
            n243 = Format Into String(format string="%02d", w340) -> (resulting string=w343:string)  [unwired: 2 in, 1 out]
            n244 = Number To Decimal String(number=w365) -> (decimal integer string=w355:string)  [unwired: 1 in]
            n245 = Number To Decimal String(number=w364) -> (decimal integer string=w354:string)  [unwired: 1 in]
            n246 = Number To Decimal String(number=w362) -> (decimal integer string=w351:string)  [unwired: 1 in]
            n247 = Number To Decimal String(number=w357) -> (decimal integer string=w352:string)  [unwired: 1 in]
            n248 = Number To Decimal String(number=w360) -> (decimal integer string=w349:string)  [unwired: 1 in]
            n249 = Concatenate Strings("MVC" ("string"), w343) -> (w339:string)
            n250 = Build Array(w339, w338, w355, w354, w353, w352, w351, w350, w349, "n/a", w333, "" ("element")) -> (w359:string[])
            n251 = call-poly <vilib>:"Write Delimited Spreadsheet.vi"("file path (dialog if empty)"=w345, "1D data"=w359, "append to file? (new file:F)"=TRUE, "delimiter (\\t)"=", " ("delimiter (\\t)")) -> ()  [unwired: 10 in, 2 out]
          }
        }
        n252 = property on="StartTrial" class="Bool (strict)"("DisabledEnum"=T3."Disabled and Grayed Out" ("Disabled")) -> ()  [unwired: 2 in, 2 out]
        n253 = property on="Reset MVC" class="Bool"("DisabledEnum"=T3."Disabled and Grayed Out" ("Disabled")) -> ()  [unwired: 2 in, 2 out]
        n254 = property on="Set Parameters" class="Bool (strict)"("DisabledEnum"=T3."Disabled and Grayed Out" ("Disabled")) -> ()  [unwired: 2 in, 2 out]
      }
      event "End Trial": Value Change {
        n255 = event-data() -> ("NewVal"=w397:bool)  [unwired: 1 in, 5 out]
        n256 = case shown="True" w397 {
          frame False {
          }
          frame True {
            n257 = local read "Trial Number"() -> (w402:dbl)
            n258 = Increment(x=w402) -> (x+1=w398:dbl)
            n259 = local write "State"(T1."No Save" ("State")) -> ()
            n260 = Format Into String(format string="%02d", w398) -> (resulting string=w401:string)  [unwired: 2 in, 1 out]
            n261 = local write "Trial Number"(w398) -> ()
            n262 = Concatenate Strings("Trial" ("string"), w401) -> (w403:string)
            n263 = property on="End Trial" class="Bool (strict)"("DisabledEnum"=T3."Disabled and Grayed Out" ("Disabled")) -> ()  [unwired: 2 in, 2 out]
            n264 = property on="Reset MVC" class="Bool"("DisabledEnum"=T3."Enabled" ("Disabled")) -> ()  [unwired: 2 in, 2 out]
            n265 = property on="Get MVC" class="Bool"("DisabledEnum"=T3."Enabled" ("Disabled")) -> ()  [unwired: 2 in, 2 out]
            n266 = property on="Set Parameters" class="Bool (strict)"("DisabledEnum"=T3."Enabled" ("Disabled")) -> ()  [unwired: 2 in, 2 out]
            n267 = property on="StartTrial" class="Bool (strict)"("DisabledEnum"=T3."Enabled" ("Disabled")) -> ()  [unwired: 2 in, 2 out]
            n268 = local write "End Trial"(FALSE ("End Trial")) -> ()
            n269 = local write "Trial Name"(w403) -> ()
          }
        }
      }
      event "StartTrial": Value Change {
        n270 = event-data() -> ("NewVal"=w411:bool)  [unwired: 1 in, 5 out]
        n271 = case shown="True" w411 {
          frame False {
          }
          frame True {
            n272 = Get Date/Time In Seconds() -> (seconds since 1Jan1904=→"TrialStartTime":timestamp)
            n273 = local write "StartTrial"(FALSE ("StartTrial")) -> ()
            n274 = local read "Data Directory"() -> (w457:path)
            n275 = local write "End Trial"(FALSE ("End Trial")) -> ()
            n276 = local read "Session Name"() -> (w456:string)
            n277 = local read "Trial Name"() -> (w439:string)
            n278 = local write "State"(T1."Trial In Progress" ("State")) -> ()
            n279 = Concatenate Strings(w439, "_FilteredData.csv" ("string")) -> (w461:string)
            n280 = Concatenate Strings(w439, "_RawData.csv" ("string")) -> (w459:string)
            n281 = Concatenate Strings(w439, "_DisplayData.csv" ("string")) -> (w463:string)
            n282 = Build Path(base path=w457, name or relative path=w456) -> (appended path=w438:path)
            n283 = property on="End Trial" class="Bool (strict)"("DisabledEnum"=T3."Enabled" ("Disabled")) -> ()  [unwired: 2 in, 2 out]
            n284 = property on="StartTrial" class="Bool (strict)"("DisabledEnum"=T3."Disabled and Grayed Out" ("Disabled")) -> ()  [unwired: 2 in, 2 out]
            n285 = property on="Reset MVC" class="Bool"("DisabledEnum"=T3."Disabled and Grayed Out" ("Disabled")) -> ()  [unwired: 2 in, 2 out]
            n286 = property on="Get MVC" class="Bool"("DisabledEnum"=T3."Disabled and Grayed Out" ("Disabled")) -> ()  [unwired: 2 in, 2 out]
            n287 = property on="Set Parameters" class="Bool (strict)"("DisabledEnum"=T3."Disabled and Grayed Out" ("Disabled")) -> ()  [unwired: 2 in, 2 out]
            n288 = Build Path(base path=w438, name or relative path="Log.csv" ("string")) -> (appended path=w422:path)
            n289 = Build Path(base path=w438, name or relative path=w461) -> (appended path=w455:path)
            n290 = Build Path(base path=w438, name or relative path=w459) -> (appended path=w454:path)
            n291 = Build Path(base path=w438, name or relative path=w463) -> (appended path=w464:path)
            n292 = local write "trial raw data"(w454) -> ()
            n293 = local write "log filepath"(w422) -> ()
            n294 = local write "trial filtered data"(w455) -> ()
            n295 = local write "trial display data"(w464) -> ()
            n296 = local read "EMG Channel To Display"() -> (w418:dbl)
            n297 = local read "EMG Channel To Display"() -> (w448:dbl)
            n298 = local read "MVC Data"() -> (w419:cluster{"queue out":refnum<queue>, dbl, dbl}[])
            n299 = local read "SecondsToAcquireMax"() -> (w447:dbl)
            n300 = local read "dispSize"() -> (w445:dbl)
            n301 = local read "lower"() -> (w442:dbl)
            n302 = Index Array(array=w419, index=w418) -> (element=w417:cluster{"queue out":refnum<queue>, dbl, dbl})
            n303 = local read "mvcSize"() -> (w446:dbl)
            n304 = local read "upper"() -> (w441:dbl)
            n305 = local read "Trial Name"() -> (w435:string)
            n306 = local read "rate"() -> (w443:dbl)
            n307 = local read "fps"() -> (w444:dbl)
            n308 = Number To Decimal String(number=w442) -> (decimal integer string=w431:string)  [unwired: 1 in]
            n309 = Number To Decimal String(number=w445) -> (decimal integer string=w429:string)  [unwired: 1 in]
            n310 = Unbundle(w417) -> (w413:dbl)  [unwired: 2 out]
            n311 = Number To Decimal String(number=w448) -> (decimal integer string=w426:string)  [unwired: 1 in]
            n312 = Get Date/Time In Seconds() -> (seconds since 1Jan1904=w421:timestamp)
            n313 = Number To Decimal String(number=w441) -> (decimal integer string=w432:string)  [unwired: 1 in]
            n314 = Number To Decimal String(number=w443) -> (decimal integer string=w430:string)  [unwired: 1 in]
            n315 = Number To Decimal String(number=w444) -> (decimal integer string=w425:string)  [unwired: 1 in]
            n316 = Number To Decimal String(number=w446) -> (decimal integer string=w428:string)  [unwired: 1 in]
            n317 = Number To Decimal String(number=w447) -> (decimal integer string=w427:string)  [unwired: 1 in]
            n318 = Format Date/Time String(time format string (%c)="%m/%d/%Y %H:%M:%S%3u", seconds (now)=w421) -> (date/time string=w416:string)  [unwired: 1 in]
            n319 = Format Value(format string="%5f", value (0)=w413) -> (output string=w412:string)  [unwired: 1 in]
            n320 = Build Array(w435, w432, w431, w430, w425, w429, w428, w427, w426, w412, w416, "Trial comment") -> (w424:string[])
            n321 = call-poly <vilib>:"Write Delimited Spreadsheet.vi"("file path (dialog if empty)"=w422, "1D data"=w424, "append to file? (new file:F)"=TRUE, "delimiter (\\t)"=", " ("delimiter (\\t)")) -> ()  [unwired: 10 in, 2 out]
          }
        }
      }
    }
  }
  n322 = Release Queue(queue=w5, error in (no error)=w1) -> ()  [unwired: 1 in, 3 out]
  n323 = while {
    stop <- w479 stop-if-true
    # "Update Display and Save Display Data"
    n324 = local read "loopTime"() -> (w478:dbl)
    n325 = local read "stop"() -> (w479:bool)
    n326 = local read "Disp Data"() -> (w482:cluster{"queue out":refnum<queue>, dbl, dbl}[])
    n327 = local read "enableSave"() -> (w469:bool)
    n328 = Wait (ms)(milliseconds to wait=w478) -> ()  [unwired: 1 out]
    n329 = local read "State"() -> (w470:T1)
    n330 = Index Array(array=w482, index="EMG Channel To Display") -> (element=w480:cluster{"queue out":refnum<queue>, dbl, dbl})
    n331 = Not Equal?(x=w470, y=T1."No Save" ("State")) -> (x != y?=w473:bool)
    n332 = Equal?(x=T1."Trial In Progress" ("State"), y=w470) -> (x = y?=w468:bool)
    n333 = Unbundle(w480) -> (w467:dbl)  [unwired: 2 out]
    "DisplayBarActivation" <- w467
    "DisplayActivation" <- w467
    n334 = And(x=w468, y=w469) -> (x .and. y?=w466:bool)
    n335 = And(x=w473, y=w469) -> (x .and. y?=→"Collecting Data":bool)
    n336 = call "BarDisplay2Var.vi"("barOrGraph"="barOrGraph", "Activation Percentage"=w467, "scale min"="Display Min", "scale max"="Display Max", "Target Percentage"="Target Percentage") -> ()  [unwired: 7 in]
    n337 = case shown="True" w466 {
      tunnel: w467 -> [_ w484]
      frame False {
      }
      frame True {
        n338 = Format Into String(w484) -> (resulting string=w489:string)  [unwired: 3 in, 1 out]
        n339 = Get Date/Time In Seconds() -> (seconds since 1Jan1904=w487:timestamp)
        n340 = Format Date/Time String(time format string (%c)="%m/%d/%Y, %H:%M:%S%3u", seconds (now)=w487) -> (date/time string=w488:string)  [unwired: 1 in]
        n341 = Build Array(w489, w488) -> (w490:string[])
        n342 = Build Array(w490) -> (w491:string[][])
        n343 = call-poly <vilib>:"Write Delimited Spreadsheet.vi"("file path (dialog if empty)"="trial display data", "2D data"=w491, "append to file? (new file:F)"=TRUE, "delimiter (\\t)"=", " ("delimiter (\\t)")) -> ()  [unwired: 10 in, 2 out]
      }
    }
  }
